vi "Start.vi"(8 "error in":errorcluster, 11 "IRunnable in":refnum<class "IRunnable.lvclass">) -> (0 "error out":errorcluster, 3 "IRunnable out":refnum<class "IRunnable.lvclass">)   [LabVIEW 2024, in "IRunnable.lvclass"]
uses:
  IRunnable.lvclass
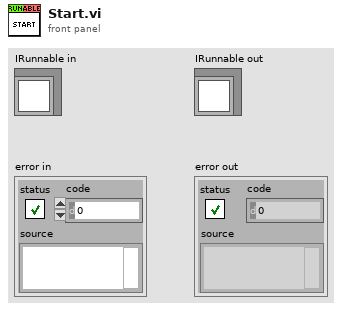
[diagram p1: front panel]
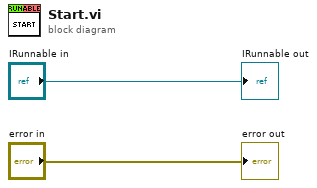
[diagram p0: block diagram]
diagram:
  "error out" <- "error in"
  "IRunnable out" <- "IRunnable in"
